vi "LoginCopia2.vi"() -> ()   [LabVIEW 2025]
uses:
  <vilib>/Utility/NIReport.llb/Report Type.ctl
  <vilib>/MakerHub/LINX/Public/Peripherals/Digital/Digital Read 1 Chan.vi
  <vilib>/MakerHub/LINX/Public/Peripherals/Digital/Digital Write 1 Chan.vi
  <vilib>/MakerHub/LINX/Public/Peripherals/Digital/Digital Read N Chans.vi
  <vilib>/MakerHub/LINX/Public/Peripherals/Digital/Digital Write N Chans.vi
  <vilib>/MakerHub/LINX/Private/Local IO/LinxDigitalRead.vi
  <vilib>/MakerHub/LINX/Public/Utilities/Check Channel.vi
  <vilib>/MakerHub/LINX/Private/Local IO/LinxDigitalWrite.vi
  <vilib>/MakerHub/LINX/Public/Utilities/Open Serial.vi
  <vilib>/addons/_office/excel.llb/Excel Easy Table (str).vi
  <vilib>/MakerHub/LINX/Private/Utilties/Generate Error.vi
  <vilib>/Utility/NIReport.llb/NI_report.lvclass
  <vilib>/MakerHub/LINX/LMH-LINX.lvlib
  <vilib>/Utility/NIReport.llb/NI_ReportGenerationCore.lvlib
  <vilib>/addons/_office/NI_ReportGenerationToolkit.lvlib
  <vilib>/Utility/NIReport.llb/Excel/NI_Excel.lvclass
panel:
  in  "stop":bool
  in  "Tab Control":enum32{"Inicio", "Sistema"}(tab)
  in  "Open Button 2":bool
  in  "Contraseña":string
  in  "Usuario":string
  out "Led 1":bool
  out "Led 2":bool
  out "Led 3":bool
  out "Led 4":bool
  out "Led 5":bool
  out "Pin2":dbl
  out "Pin3":dbl
  out "Pin4":dbl
  out "Pin5":dbl
  out "Pin6":dbl
  in  "Puerto Serial":refnum<visa-resource-name>="N/A"
  in  "Secuencia":dbl
  out "Contenido":dbl
  in  "Detener":bool
  in  "Registro Excel":path
  in  "stop 4":bool
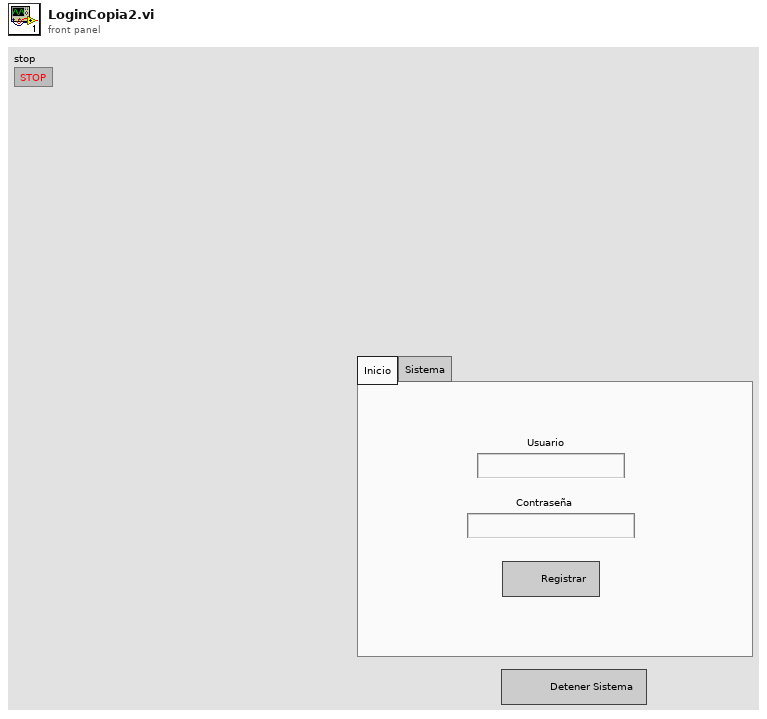
[diagram p1: front panel]
types:
  T1 = typedef "NI_ReportGenerationCore.lvlib/Report Type.ctl" = enum16{"HTML", "Word", "Excel"}
  T2 = typedef "LMH-LINX.lvlib/LINX Ref.ctl" = cluster{"IO":T3, "Interface":T4, "LINX Device Config":T5}
  T3 = typedef "LMH-LINX.lvlib/Platform.ctl" = enum16{"Remote", "Local"}
  T4 = typedef "LMH-LINX.lvlib/Interface.ctl" = enum16{"Serial", "TCP"}
  T5 = typedef "LMH-LINX.lvlib/Device.lvlib/LINX Device Config.ctl" = cluster{"Interface":T4, "COM Port":refnum<visa-resource-name>, "TCP Configuration":T6, "Device Family":u8, "Device ID":u8, "Device Name":string, "TCP Ref":refnum<k5>, "Channels":T7}
  T6 = typedef "LMH-LINX.lvlib/Device.lvlib/TCP Config.ctl" = cluster{"IP Address":string, "Port":u16}
  T7 = typedef "LMH-LINX.lvlib/Channels.ctl" = cluster{"DI":u8[], "DO":u8[], "AI":u8[], "AO":u8[], "PWM":u8[], "QE":u8[], "UART":u8[], "I2C 2":u8[], "SPI":u8[], "CAN":u8[], "Servo":u8[], "AI Ref (V)":dbl, "AI Resolution (Bits)":u8, "AO Ref (V)":dbl, "AO Resolution (Bits)":u8}
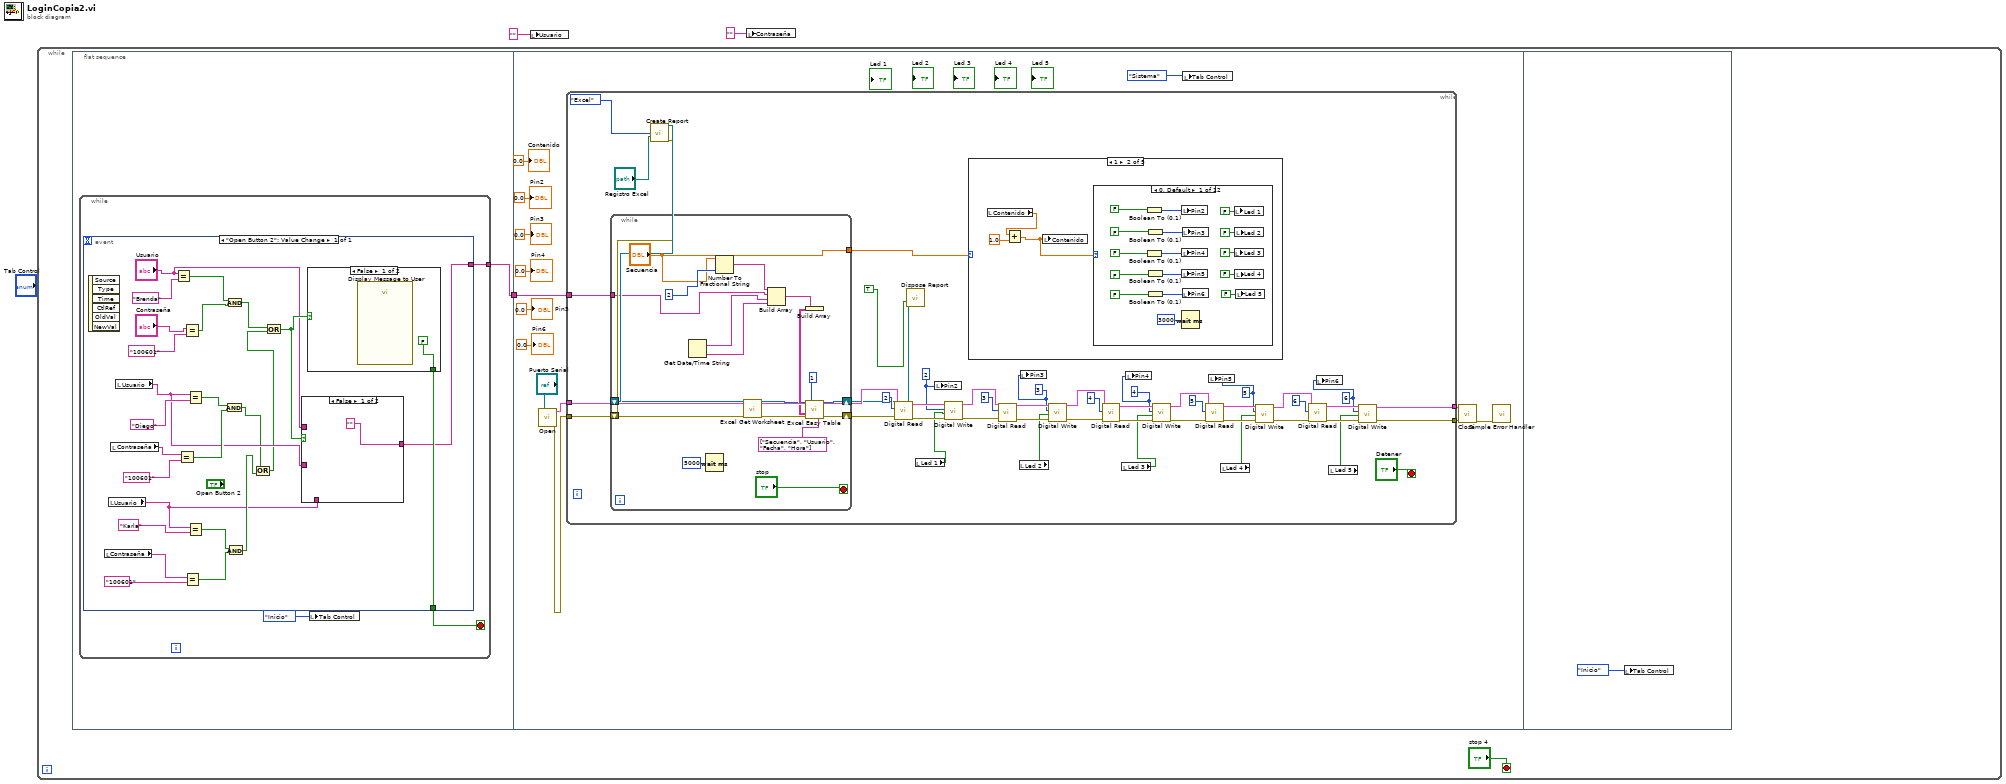
[diagram p0: block diagram]
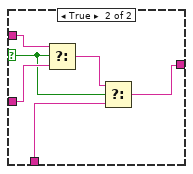
[diagram p2: hidden frame]
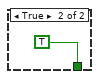
[diagram p3: hidden frame]
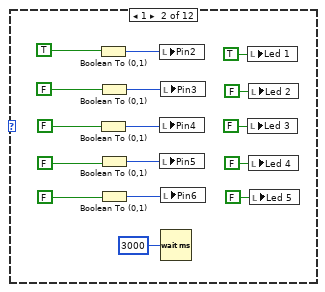
[diagram p5: hidden frame]
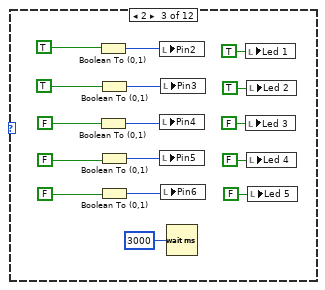
[diagram p6: hidden frame]
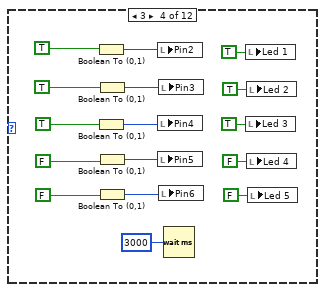
[diagram p7: hidden frame]
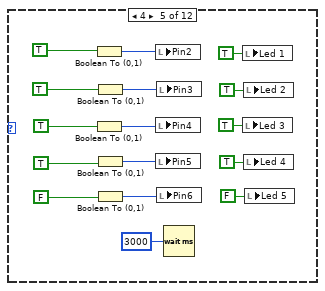
[diagram p8: hidden frame]
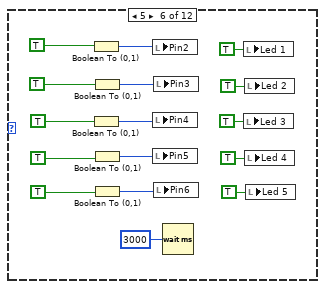
[diagram p9: hidden frame]
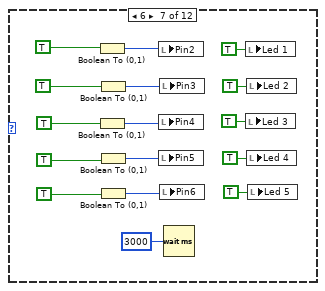
[diagram p10: hidden frame]
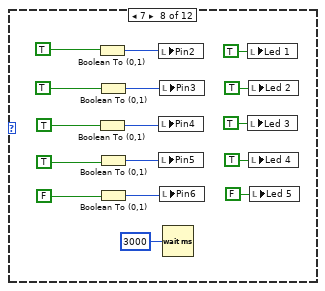
[diagram p11: hidden frame]
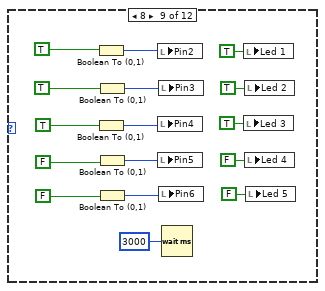
[diagram p12: hidden frame]
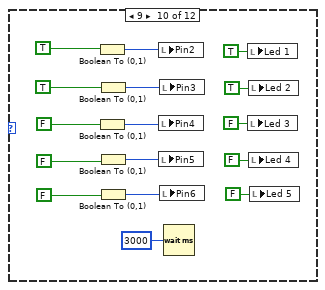
[diagram p13: hidden frame]
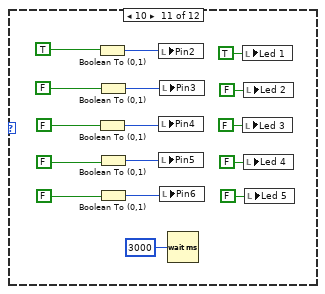
[diagram p14: hidden frame]
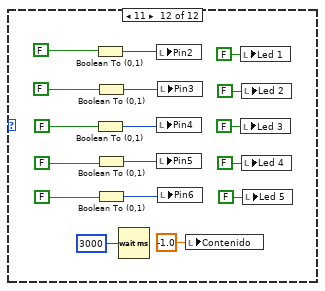
[diagram p15: hidden frame]
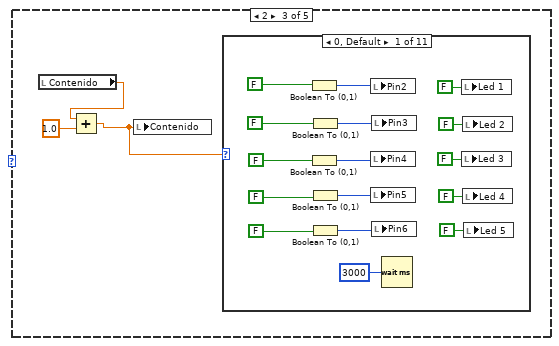
[diagram p16: hidden frame]
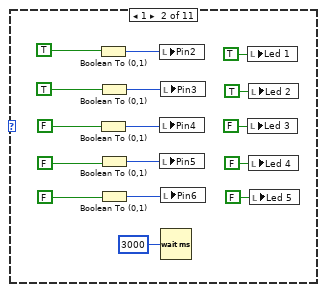
[diagram p17: hidden frame]
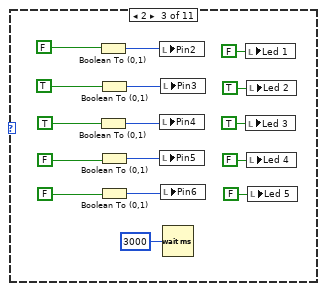
[diagram p18: hidden frame]
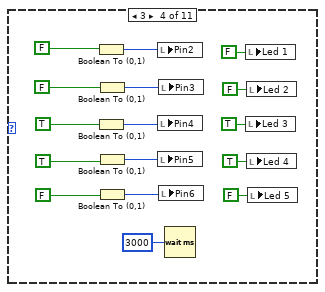
[diagram p19: hidden frame]
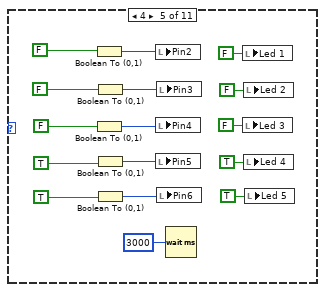
[diagram p20: hidden frame]
diagram:
  n1 = while {
    stop <- "stop 4" stop-if-true
    n2 = flat-sequence {
      tunnel: [w5] -> w3
      tunnel: w3 -> [w43]
      frame #0 {
        n3 = while {
          tunnel: [w6] -> w5
          stop <- w8 stop-if-true
          n4 = event shown="[0] \"Open Button 2\": Value Change" {
            selector: _ -> [_]
            dyn-events: _ -> [_]
            timeout: _ -> [_]
            tunnel: [w33] -> w8
            tunnel: [w18] -> w6
            event "Open Button 2": Value Change {
              n5 = event-data() -> ()  [unwired: 1 in, 6 out]
              n6 = local read "Contraseña"() -> (w16:string)
              n7 = local read "Usuario"() -> (w9:string)
              n8 = local read "Contraseña"() -> (w27:string)
              n9 = local read "Usuario"() -> (w19:string)
              n10 = Equal?(x="Usuario", y="Brenda") -> (x = y?=w23:bool)
              n11 = Equal?(x=w27, y="100601") -> (x = y?=w25:bool)
              n12 = Equal?(x="Contraseña", y="100601") -> (x = y?=w30:bool)
              n13 = Equal?(x=w16, y="100601") -> (x = y?=w13:bool)
              n14 = Equal?(x=w19, y="Diego") -> (x = y?=w26:bool)
              n15 = Equal?(x=w9, y="Karla") -> (x = y?=w14:bool)
              n16 = And(x=w26, y=w25) -> (x .and. y?=w11:bool)
              n17 = And(x=w23, y=w30) -> (x .and. y?=w24:bool)
              n18 = And(x=w14, y=w13) -> (x .and. y?=w12:bool)
              n19 = Or(x=w11, y=w12) -> (x .or. y?=w10:bool)
              n20 = Or(x=w24, y=w10) -> (x .or. y?=w21:bool)
              n21 = case shown="False" w21 {
                selector: w21 -> [_ w35]
                tunnel: "Usuario" -> [_ w40]
                tunnel: w19 -> [_ w39]
                tunnel: ["" ("y") w36] -> w18
                tunnel: w9 -> [_ w38]
                frame False {
                }
                frame True {
                  n22 = Select(t=w40, s=w35, f=w39) -> (s? t:f=w37:string)
                  n23 = Select(t=w37, s=w35, f=w38) -> (s? t:f=w36:string)
                }
              }
              n24 = case shown="False" w21 {
                tunnel: [FALSE TRUE] -> w33
                frame False {
                  n25 = call "Display Message to User"() -> ()  [unwired: 10 in, 2 out]
                }
                frame True {
                }
              }
            }
          }
          n26 = local write "Tab Control"(enum32{"Inicio", "Sistema"}."Inicio" ("Tab Control")) -> ()
        }
      }
      frame #1 {
        n27 = call-poly <vilib>:"Open.vi"("Serial Port"="Puerto Serial") -> ("Error Out"=w45:errorcluster, "LINX Resource"=w46:T2)  [unwired: 8 in, 1 out]
        n28 = while {
          tunnel: [w70] -> w48
          tunnel: [w69] -> w47
          tunnel: w46 -> [w68]
          tunnel: w45 -> [w67]
          tunnel: w43 -> [w57]
          stop <- "Detener" stop-if-true
          w71 = u8 6 ("DO Channel")
          w74 = u8 5 ("DO Channel")
          w75 = u8 4 ("DO Channel")
          w80 = u8 3 ("DO Channel")
          w78 = u8 2 ("DO Channel")
          n29 = call <vilib>:"Create Report.vi"("report type"=Report_Type."Excel", "template (empty)"="Registro Excel") -> ("report out"=w63:refnum<class "NI_report.lvclass">, "error out"=w62:errorcluster)  [unwired: 12 in]
          n30 = while {
            shift-right: [w112] -> w61
            shift-left: w63 -> [w116]
            shift-right: [w111] -> w60
            shift-left: w62 -> [w114]
            tunnel: ["Secuencia"] -> w58
            tunnel: w57 -> [w106]
            stop <- "stop" stop-if-true
            n31 = Get Date/Time String() -> (date string=w105:string, time string=w104:string)  [unwired: 3 in]
            n32 = Wait (ms)(milliseconds to wait=u32 5000) -> ()  [unwired: 1 out]
            n33 = Number To Fractional String(number="Secuencia", precision (6)=i16 2) -> (F-format string=w120:string)  [unwired: 2 in]
            n34 = call <vilib>:"Excel Get Worksheet.vi"("report in"=w116, "error in (no error)"=w114) -> ("report out"=w115:refnum<class "NI_report.lvclass">, "error out"=w113:errorcluster)  [unwired: 12 in]
            n35 = Build Array(w120, w106, w105, w104) -> (w119:string[])
            n36 = Build Array(w119) -> (w118:string[][])
            n37 = call-poly <vilib>:"Excel Easy Table.vi"("report in"=w115, "iteration"=1, "text data"=w118, "error in (no error)"=w113, "column headers"=string[] ["Secuencia", "Usuario", "Fecha", "Hora"]) -> ("report out"=w112:refnum<class "NI_report.lvclass">, "error out"=w111:errorcluster)  [unwired: 6 in, 3 out]
          }
          n38 = call-poly <vilib>:"Digital Read.vi"("Error In"=w67, "DI Channel"=u8 2, "LINX Resource"=w68) -> ("Error Out"=w89:errorcluster, "LINX Resource"=w98:T2)  [unwired: 6 in, 1 out]
          n39 = call-dynamic "Dispose Report.vi"("report in"=w61, "save changes? (F)"=TRUE, "error in (no error)"=w60) -> ()  [unwired: 12 in, 1 out]
          n40 = local read "Led 1"() -> (w79:bool)
          n41 = local write "Pin2"(w78) -> ()
          n42 = call-poly <vilib>:"Digital Write.vi"("Error In"=w89, "Output Value"=w79, "DO Channel"=w78, "LINX Resource"=w98) -> ("Error Out"=w88:errorcluster, "LINX Resource"=w97:T2)  [unwired: 6 in]
          n43 = case shown="1" w58 {
            frame 0, Default {
            }
            frame 1 {
              n44 = local read "Contenido"() -> (w123:dbl)
              n45 = Add(x=w123, y=1.0) -> (x+y=w122:dbl)
              n46 = local write "Contenido"(w122) -> ()
              n47 = case shown="0, Default" w122 {
                frame 0, Default {
                  n48 = Boolean To (0,1)(Boolean=FALSE) -> (0, 1=w140:i16)
                  n49 = Boolean To (0,1)(Boolean=FALSE) -> (0, 1=w138:i16)
                  n50 = Boolean To (0,1)(Boolean=FALSE) -> (0, 1=w139:i16)
                  n51 = Boolean To (0,1)(Boolean=FALSE) -> (0, 1=w137:i16)
                  n52 = Boolean To (0,1)(Boolean=FALSE) -> (0, 1=w136:i16)
                  n53 = local write "Pin2"(w140) -> ()
                  n54 = local write "Pin4"(w138) -> ()
                  n55 = local write "Pin5"(w137) -> ()
                  n56 = Wait (ms)(milliseconds to wait=u32 3000 ("millisecond timer value")) -> ()  [unwired: 1 out]
                  n57 = local write "Pin3"(w139) -> ()
                  n58 = local write "Pin6"(w136) -> ()
                  n59 = local write "Led 1"(FALSE ("Led 1")) -> ()
                  n60 = local write "Led 3"(FALSE ("Led 3")) -> ()
                  n61 = local write "Led 2"(FALSE ("Led 2")) -> ()
                  n62 = local write "Led 4"(FALSE ("Led 4")) -> ()
                  n63 = local write "Led 5"(FALSE ("Led 5")) -> ()
                }
                frame 1 {
                  n64 = Boolean To (0,1)(Boolean=TRUE) -> (0, 1=w155:i16)
                  n65 = Boolean To (0,1)(Boolean=FALSE) -> (0, 1=w151:i16)
                  n66 = Boolean To (0,1)(Boolean=FALSE) -> (0, 1=w153:i16)
                  n67 = Boolean To (0,1)(Boolean=FALSE) -> (0, 1=w149:i16)
                  n68 = Boolean To (0,1)(Boolean=FALSE) -> (0, 1=w147:i16)
                  n69 = local write "Pin2"(w155) -> ()
                  n70 = local write "Pin4"(w151) -> ()
                  n71 = local write "Pin5"(w149) -> ()
                  n72 = local write "Pin3"(w153) -> ()
                  n73 = local write "Pin6"(w147) -> ()
                  n74 = Wait (ms)(milliseconds to wait=u32 3000 ("millisecond timer value")) -> ()  [unwired: 1 out]
                  n75 = local write "Led 1"(TRUE ("Led 1")) -> ()
                  n76 = local write "Led 3"(FALSE ("Led 3")) -> ()
                  n77 = local write "Led 2"(FALSE ("Led 2")) -> ()
                  n78 = local write "Led 4"(FALSE ("Led 4")) -> ()
                  n79 = local write "Led 5"(FALSE ("Led 5")) -> ()
                }
                frame 2 {
                  n80 = Boolean To (0,1)(Boolean=TRUE) -> (0, 1=w172:i16)
                  n81 = Boolean To (0,1)(Boolean=FALSE) -> (0, 1=w170:i16)
                  n82 = Boolean To (0,1)(Boolean=TRUE) -> (0, 1=w171:i16)
                  n83 = Boolean To (0,1)(Boolean=FALSE) -> (0, 1=w169:i16)
                  n84 = Boolean To (0,1)(Boolean=FALSE) -> (0, 1=w168:i16)
                  n85 = local write "Pin2"(w172) -> ()
                  n86 = local write "Pin4"(w170) -> ()
                  n87 = local write "Pin5"(w169) -> ()
                  n88 = local write "Pin3"(w171) -> ()
                  n89 = local write "Pin6"(w168) -> ()
                  n90 = Wait (ms)(milliseconds to wait=u32 3000 ("millisecond timer value")) -> ()  [unwired: 1 out]
                  n91 = local write "Led 1"(TRUE ("Led 1")) -> ()
                  n92 = local write "Led 3"(FALSE ("Led 3")) -> ()
                  n93 = local write "Led 2"(TRUE ("Led 2")) -> ()
                  n94 = local write "Led 4"(FALSE ("Led 4")) -> ()
                  n95 = local write "Led 5"(FALSE ("Led 5")) -> ()
                }
                frame 3 {
                  n96 = Boolean To (0,1)(Boolean=TRUE) -> (0, 1=w188:i16)
                  n97 = Boolean To (0,1)(Boolean=TRUE) -> (0, 1=w186:i16)
                  n98 = Boolean To (0,1)(Boolean=TRUE) -> (0, 1=w187:i16)
                  n99 = Boolean To (0,1)(Boolean=FALSE) -> (0, 1=w185:i16)
                  n100 = Boolean To (0,1)(Boolean=FALSE) -> (0, 1=w184:i16)
                  n101 = local write "Pin2"(w188) -> ()
                  n102 = local write "Pin4"(w186) -> ()
                  n103 = local write "Pin5"(w185) -> ()
                  n104 = local write "Pin3"(w187) -> ()
                  n105 = local write "Pin6"(w184) -> ()
                  n106 = Wait (ms)(milliseconds to wait=u32 3000 ("millisecond timer value")) -> ()  [unwired: 1 out]
                  n107 = local write "Led 1"(TRUE ("Led 1")) -> ()
                  n108 = local write "Led 3"(TRUE ("Led 3")) -> ()
                  n109 = local write "Led 2"(TRUE ("Led 2")) -> ()
                  n110 = local write "Led 4"(FALSE ("Led 4")) -> ()
                  n111 = local write "Led 5"(FALSE ("Led 5")) -> ()
                }
                frame 4 {
                  n112 = Boolean To (0,1)(Boolean=TRUE) -> (0, 1=w204:i16)
                  n113 = Boolean To (0,1)(Boolean=TRUE) -> (0, 1=w202:i16)
                  n114 = Boolean To (0,1)(Boolean=TRUE) -> (0, 1=w203:i16)
                  n115 = Boolean To (0,1)(Boolean=TRUE) -> (0, 1=w201:i16)
                  n116 = Boolean To (0,1)(Boolean=FALSE) -> (0, 1=w200:i16)
                  n117 = local write "Pin2"(w204) -> ()
                  n118 = local write "Pin4"(w202) -> ()
                  n119 = local write "Pin5"(w201) -> ()
                  n120 = local write "Pin3"(w203) -> ()
                  n121 = local write "Pin6"(w200) -> ()
                  n122 = Wait (ms)(milliseconds to wait=u32 3000 ("millisecond timer value")) -> ()  [unwired: 1 out]
                  n123 = local write "Led 1"(TRUE ("Led 1")) -> ()
                  n124 = local write "Led 3"(TRUE ("Led 3")) -> ()
                  n125 = local write "Led 2"(TRUE ("Led 2")) -> ()
                  n126 = local write "Led 4"(TRUE ("Led 4")) -> ()
                  n127 = local write "Led 5"(FALSE ("Led 5")) -> ()
                }
                frame 5 {
                  n128 = Boolean To (0,1)(Boolean=TRUE) -> (0, 1=w220:i16)
                  n129 = Boolean To (0,1)(Boolean=TRUE) -> (0, 1=w218:i16)
                  n130 = Boolean To (0,1)(Boolean=TRUE) -> (0, 1=w219:i16)
                  n131 = Boolean To (0,1)(Boolean=TRUE) -> (0, 1=w217:i16)
                  n132 = Boolean To (0,1)(Boolean=TRUE) -> (0, 1=w216:i16)
                  n133 = local write "Pin2"(w220) -> ()
                  n134 = local write "Pin4"(w218) -> ()
                  n135 = local write "Pin5"(w217) -> ()
                  n136 = local write "Pin3"(w219) -> ()
                  n137 = local write "Pin6"(w216) -> ()
                  n138 = Wait (ms)(milliseconds to wait=u32 3000 ("millisecond timer value")) -> ()  [unwired: 1 out]
                  n139 = local write "Led 1"(TRUE ("Led 1")) -> ()
                  n140 = local write "Led 3"(TRUE ("Led 3")) -> ()
                  n141 = local write "Led 2"(TRUE ("Led 2")) -> ()
                  n142 = local write "Led 4"(TRUE ("Led 4")) -> ()
                  n143 = local write "Led 5"(TRUE ("Led 5")) -> ()
                }
                frame 6 {
                  n144 = Boolean To (0,1)(Boolean=TRUE) -> (0, 1=w236:i16)
                  n145 = Boolean To (0,1)(Boolean=TRUE) -> (0, 1=w234:i16)
                  n146 = Boolean To (0,1)(Boolean=TRUE) -> (0, 1=w235:i16)
                  n147 = Boolean To (0,1)(Boolean=TRUE) -> (0, 1=w233:i16)
                  n148 = Boolean To (0,1)(Boolean=TRUE) -> (0, 1=w232:i16)
                  n149 = local write "Pin2"(w236) -> ()
                  n150 = local write "Pin4"(w234) -> ()
                  n151 = local write "Pin5"(w233) -> ()
                  n152 = local write "Pin3"(w235) -> ()
                  n153 = local write "Pin6"(w232) -> ()
                  n154 = Wait (ms)(milliseconds to wait=u32 3000 ("millisecond timer value")) -> ()  [unwired: 1 out]
                  n155 = local write "Led 1"(TRUE ("Led 1")) -> ()
                  n156 = local write "Led 3"(TRUE ("Led 3")) -> ()
                  n157 = local write "Led 2"(TRUE ("Led 2")) -> ()
                  n158 = local write "Led 4"(TRUE ("Led 4")) -> ()
                  n159 = local write "Led 5"(TRUE ("Led 5")) -> ()
                }
                frame 7 {
                  n160 = Boolean To (0,1)(Boolean=TRUE) -> (0, 1=w252:i16)
                  n161 = Boolean To (0,1)(Boolean=TRUE) -> (0, 1=w250:i16)
                  n162 = Boolean To (0,1)(Boolean=TRUE) -> (0, 1=w251:i16)
                  n163 = Boolean To (0,1)(Boolean=TRUE) -> (0, 1=w249:i16)
                  n164 = Boolean To (0,1)(Boolean=FALSE) -> (0, 1=w248:i16)
                  n165 = local write "Pin2"(w252) -> ()
                  n166 = local write "Pin4"(w250) -> ()
                  n167 = local write "Pin5"(w249) -> ()
                  n168 = local write "Pin3"(w251) -> ()
                  n169 = local write "Pin6"(w248) -> ()
                  n170 = Wait (ms)(milliseconds to wait=u32 3000 ("millisecond timer value")) -> ()  [unwired: 1 out]
                  n171 = local write "Led 1"(TRUE ("Led 1")) -> ()
                  n172 = local write "Led 3"(TRUE ("Led 3")) -> ()
                  n173 = local write "Led 2"(TRUE ("Led 2")) -> ()
                  n174 = local write "Led 4"(TRUE ("Led 4")) -> ()
                  n175 = local write "Led 5"(FALSE ("Led 5")) -> ()
                }
                frame 8 {
                  n176 = Boolean To (0,1)(Boolean=TRUE) -> (0, 1=w268:i16)
                  n177 = Boolean To (0,1)(Boolean=TRUE) -> (0, 1=w266:i16)
                  n178 = Boolean To (0,1)(Boolean=TRUE) -> (0, 1=w267:i16)
                  n179 = Boolean To (0,1)(Boolean=FALSE) -> (0, 1=w265:i16)
                  n180 = Boolean To (0,1)(Boolean=FALSE) -> (0, 1=w264:i16)
                  n181 = local write "Pin2"(w268) -> ()
                  n182 = local write "Pin4"(w266) -> ()
                  n183 = local write "Pin5"(w265) -> ()
                  n184 = local write "Pin3"(w267) -> ()
                  n185 = local write "Pin6"(w264) -> ()
                  n186 = Wait (ms)(milliseconds to wait=u32 3000 ("millisecond timer value")) -> ()  [unwired: 1 out]
                  n187 = local write "Led 1"(TRUE ("Led 1")) -> ()
                  n188 = local write "Led 3"(TRUE ("Led 3")) -> ()
                  n189 = local write "Led 2"(TRUE ("Led 2")) -> ()
                  n190 = local write "Led 4"(FALSE ("Led 4")) -> ()
                  n191 = local write "Led 5"(FALSE ("Led 5")) -> ()
                }
                frame 9 {
                  n192 = Boolean To (0,1)(Boolean=TRUE) -> (0, 1=w284:i16)
                  n193 = Boolean To (0,1)(Boolean=FALSE) -> (0, 1=w282:i16)
                  n194 = Boolean To (0,1)(Boolean=TRUE) -> (0, 1=w283:i16)
                  n195 = Boolean To (0,1)(Boolean=FALSE) -> (0, 1=w281:i16)
                  n196 = Boolean To (0,1)(Boolean=FALSE) -> (0, 1=w280:i16)
                  n197 = local write "Pin2"(w284) -> ()
                  n198 = local write "Pin4"(w282) -> ()
                  n199 = local write "Pin5"(w281) -> ()
                  n200 = local write "Pin3"(w283) -> ()
                  n201 = local write "Pin6"(w280) -> ()
                  n202 = Wait (ms)(milliseconds to wait=u32 3000 ("millisecond timer value")) -> ()  [unwired: 1 out]
                  n203 = local write "Led 1"(TRUE ("Led 1")) -> ()
                  n204 = local write "Led 3"(FALSE ("Led 3")) -> ()
                  n205 = local write "Led 2"(TRUE ("Led 2")) -> ()
                  n206 = local write "Led 4"(FALSE ("Led 4")) -> ()
                  n207 = local write "Led 5"(FALSE ("Led 5")) -> ()
                }
                frame 10 {
                  n208 = Boolean To (0,1)(Boolean=TRUE) -> (0, 1=w300:i16)
                  n209 = Boolean To (0,1)(Boolean=FALSE) -> (0, 1=w298:i16)
                  n210 = Boolean To (0,1)(Boolean=FALSE) -> (0, 1=w299:i16)
                  n211 = Boolean To (0,1)(Boolean=FALSE) -> (0, 1=w297:i16)
                  n212 = Boolean To (0,1)(Boolean=FALSE) -> (0, 1=w296:i16)
                  n213 = local write "Pin2"(w300) -> ()
                  n214 = local write "Pin4"(w298) -> ()
                  n215 = local write "Pin5"(w297) -> ()
                  n216 = local write "Pin3"(w299) -> ()
                  n217 = local write "Pin6"(w296) -> ()
                  n218 = Wait (ms)(milliseconds to wait=u32 3000 ("millisecond timer value")) -> ()  [unwired: 1 out]
                  n219 = local write "Led 1"(TRUE ("Led 1")) -> ()
                  n220 = local write "Led 3"(FALSE ("Led 3")) -> ()
                  n221 = local write "Led 2"(FALSE ("Led 2")) -> ()
                  n222 = local write "Led 4"(FALSE ("Led 4")) -> ()
                  n223 = local write "Led 5"(FALSE ("Led 5")) -> ()
                }
                frame 11 {
                  n224 = Boolean To (0,1)(Boolean=FALSE) -> (0, 1=w317:i16)
                  n225 = Boolean To (0,1)(Boolean=FALSE) -> (0, 1=w315:i16)
                  n226 = Boolean To (0,1)(Boolean=FALSE) -> (0, 1=w316:i16)
                  n227 = Boolean To (0,1)(Boolean=FALSE) -> (0, 1=w314:i16)
                  n228 = Boolean To (0,1)(Boolean=FALSE) -> (0, 1=w313:i16)
                  n229 = Wait (ms)(milliseconds to wait=u32 3000 ("millisecond timer value")) -> ()  [unwired: 1 out]
                  n230 = local write "Pin2"(w317) -> ()
                  n231 = local write "Pin4"(w315) -> ()
                  n232 = local write "Pin5"(w314) -> ()
                  n233 = local write "Pin3"(w316) -> ()
                  n234 = local write "Pin6"(w313) -> ()
                  n235 = local write "Contenido"(-1.0 ("Contenido")) -> ()
                  n236 = local write "Led 1"(FALSE ("Led 1")) -> ()
                  n237 = local write "Led 3"(FALSE ("Led 3")) -> ()
                  n238 = local write "Led 2"(FALSE ("Led 2")) -> ()
                  n239 = local write "Led 4"(FALSE ("Led 4")) -> ()
                  n240 = local write "Led 5"(FALSE ("Led 5")) -> ()
                }
              }
            }
            frame 2 {
              n241 = local read "Contenido"() -> (w320:dbl)
              n242 = Add(x=w320, y=1.0) -> (x+y=w319:dbl)
              n243 = local write "Contenido"(w319) -> ()
              n244 = case shown="0, Default" w319 {
                frame 0, Default {
                  n245 = Boolean To (0,1)(Boolean=FALSE) -> (0, 1=w336:i16)
                  n246 = Boolean To (0,1)(Boolean=FALSE) -> (0, 1=w334:i16)
                  n247 = Boolean To (0,1)(Boolean=FALSE) -> (0, 1=w335:i16)
                  n248 = Boolean To (0,1)(Boolean=FALSE) -> (0, 1=w333:i16)
                  n249 = Boolean To (0,1)(Boolean=FALSE) -> (0, 1=w332:i16)
                  n250 = local write "Pin2"(w336) -> ()
                  n251 = local write "Pin4"(w334) -> ()
                  n252 = local write "Pin5"(w333) -> ()
                  n253 = local write "Pin3"(w335) -> ()
                  n254 = local write "Pin6"(w332) -> ()
                  n255 = Wait (ms)(milliseconds to wait=u32 3000 ("millisecond timer value")) -> ()  [unwired: 1 out]
                  n256 = local write "Led 1"(FALSE ("Led 1")) -> ()
                  n257 = local write "Led 3"(FALSE ("Led 3")) -> ()
                  n258 = local write "Led 2"(FALSE ("Led 2")) -> ()
                  n259 = local write "Led 4"(FALSE ("Led 4")) -> ()
                  n260 = local write "Led 5"(FALSE ("Led 5")) -> ()
                }
                frame 1 {
                  n261 = Boolean To (0,1)(Boolean=TRUE) -> (0, 1=w351:i16)
                  n262 = Boolean To (0,1)(Boolean=FALSE) -> (0, 1=w347:i16)
                  n263 = Boolean To (0,1)(Boolean=TRUE) -> (0, 1=w349:i16)
                  n264 = Boolean To (0,1)(Boolean=FALSE) -> (0, 1=w345:i16)
                  n265 = Boolean To (0,1)(Boolean=FALSE) -> (0, 1=w343:i16)
                  n266 = local write "Pin2"(w351) -> ()
                  n267 = local write "Pin4"(w347) -> ()
                  n268 = local write "Pin5"(w345) -> ()
                  n269 = local write "Pin3"(w349) -> ()
                  n270 = local write "Pin6"(w343) -> ()
                  n271 = Wait (ms)(milliseconds to wait=u32 3000 ("millisecond timer value")) -> ()  [unwired: 1 out]
                  n272 = local write "Led 1"(TRUE ("Led 1")) -> ()
                  n273 = local write "Led 3"(FALSE ("Led 3")) -> ()
                  n274 = local write "Led 2"(TRUE ("Led 2")) -> ()
                  n275 = local write "Led 4"(FALSE ("Led 4")) -> ()
                  n276 = local write "Led 5"(FALSE ("Led 5")) -> ()
                }
                frame 2 {
                  n277 = Boolean To (0,1)(Boolean=FALSE) -> (0, 1=w368:i16)
                  n278 = Boolean To (0,1)(Boolean=TRUE) -> (0, 1=w366:i16)
                  n279 = Boolean To (0,1)(Boolean=TRUE) -> (0, 1=w367:i16)
                  n280 = Boolean To (0,1)(Boolean=FALSE) -> (0, 1=w365:i16)
                  n281 = Boolean To (0,1)(Boolean=FALSE) -> (0, 1=w364:i16)
                  n282 = local write "Pin2"(w368) -> ()
                  n283 = local write "Pin4"(w366) -> ()
                  n284 = local write "Pin5"(w365) -> ()
                  n285 = local write "Pin3"(w367) -> ()
                  n286 = local write "Pin6"(w364) -> ()
                  n287 = Wait (ms)(milliseconds to wait=u32 3000 ("millisecond timer value")) -> ()  [unwired: 1 out]
                  n288 = local write "Led 1"(FALSE ("Led 1")) -> ()
                  n289 = local write "Led 3"(TRUE ("Led 3")) -> ()
                  n290 = local write "Led 2"(TRUE ("Led 2")) -> ()
                  n291 = local write "Led 4"(FALSE ("Led 4")) -> ()
                  n292 = local write "Led 5"(FALSE ("Led 5")) -> ()
                }
                frame 3 {
                  n293 = Boolean To (0,1)(Boolean=FALSE) -> (0, 1=w384:i16)
                  n294 = Boolean To (0,1)(Boolean=TRUE) -> (0, 1=w382:i16)
                  n295 = Boolean To (0,1)(Boolean=FALSE) -> (0, 1=w383:i16)
                  n296 = Boolean To (0,1)(Boolean=TRUE) -> (0, 1=w381:i16)
                  n297 = Boolean To (0,1)(Boolean=FALSE) -> (0, 1=w380:i16)
                  n298 = local write "Pin2"(w384) -> ()
                  n299 = local write "Pin4"(w382) -> ()
                  n300 = local write "Pin5"(w381) -> ()
                  n301 = local write "Pin3"(w383) -> ()
                  n302 = local write "Pin6"(w380) -> ()
                  n303 = Wait (ms)(milliseconds to wait=u32 3000 ("millisecond timer value")) -> ()  [unwired: 1 out]
                  n304 = local write "Led 1"(FALSE ("Led 1")) -> ()
                  n305 = local write "Led 3"(TRUE ("Led 3")) -> ()
                  n306 = local write "Led 2"(FALSE ("Led 2")) -> ()
                  n307 = local write "Led 4"(TRUE ("Led 4")) -> ()
                  n308 = local write "Led 5"(FALSE ("Led 5")) -> ()
                }
                frame 4 {
                  n309 = Boolean To (0,1)(Boolean=FALSE) -> (0, 1=w400:i16)
                  n310 = Boolean To (0,1)(Boolean=FALSE) -> (0, 1=w398:i16)
                  n311 = Boolean To (0,1)(Boolean=FALSE) -> (0, 1=w399:i16)
                  n312 = Boolean To (0,1)(Boolean=TRUE) -> (0, 1=w397:i16)
                  n313 = Boolean To (0,1)(Boolean=TRUE) -> (0, 1=w396:i16)
                  n314 = local write "Pin2"(w400) -> ()
                  n315 = local write "Pin4"(w398) -> ()
                  n316 = local write "Pin5"(w397) -> ()
                  n317 = local write "Pin3"(w399) -> ()
                  n318 = local write "Pin6"(w396) -> ()
                  n319 = Wait (ms)(milliseconds to wait=u32 3000 ("millisecond timer value")) -> ()  [unwired: 1 out]
                  n320 = local write "Led 1"(FALSE ("Led 1")) -> ()
                  n321 = local write "Led 3"(FALSE ("Led 3")) -> ()
                  n322 = local write "Led 2"(FALSE ("Led 2")) -> ()
                  n323 = local write "Led 4"(TRUE ("Led 4")) -> ()
                  n324 = local write "Led 5"(TRUE ("Led 5")) -> ()
                }
                frame 5 {
                  n325 = Boolean To (0,1)(Boolean=FALSE) -> (0, 1=w416:i16)
                  n326 = Boolean To (0,1)(Boolean=FALSE) -> (0, 1=w414:i16)
                  n327 = Boolean To (0,1)(Boolean=FALSE) -> (0, 1=w415:i16)
                  n328 = Boolean To (0,1)(Boolean=FALSE) -> (0, 1=w413:i16)
                  n329 = Boolean To (0,1)(Boolean=FALSE) -> (0, 1=w412:i16)
                  n330 = local write "Pin2"(w416) -> ()
                  n331 = local write "Pin4"(w414) -> ()
                  n332 = local write "Pin5"(w413) -> ()
                  n333 = local write "Pin3"(w415) -> ()
                  n334 = local write "Pin6"(w412) -> ()
                  n335 = Wait (ms)(milliseconds to wait=u32 3000 ("millisecond timer value")) -> ()  [unwired: 1 out]
                  n336 = local write "Led 1"(FALSE ("Led 1")) -> ()
                  n337 = local write "Led 3"(FALSE ("Led 3")) -> ()
                  n338 = local write "Led 2"(FALSE ("Led 2")) -> ()
                  n339 = local write "Led 4"(FALSE ("Led 4")) -> ()
                  n340 = local write "Led 5"(FALSE ("Led 5")) -> ()
                }
                frame 6 {
                  n341 = Boolean To (0,1)(Boolean=FALSE) -> (0, 1=w432:i16)
                  n342 = Boolean To (0,1)(Boolean=FALSE) -> (0, 1=w430:i16)
                  n343 = Boolean To (0,1)(Boolean=FALSE) -> (0, 1=w431:i16)
                  n344 = Boolean To (0,1)(Boolean=TRUE) -> (0, 1=w429:i16)
                  n345 = Boolean To (0,1)(Boolean=TRUE) -> (0, 1=w428:i16)
                  n346 = local write "Pin2"(w432) -> ()
                  n347 = local write "Pin4"(w430) -> ()
                  n348 = local write "Pin5"(w429) -> ()
                  n349 = local write "Pin3"(w431) -> ()
                  n350 = local write "Pin6"(w428) -> ()
                  n351 = Wait (ms)(milliseconds to wait=u32 3000 ("millisecond timer value")) -> ()  [unwired: 1 out]
                  n352 = local write "Led 1"(FALSE ("Led 1")) -> ()
                  n353 = local write "Led 3"(FALSE ("Led 3")) -> ()
                  n354 = local write "Led 2"(FALSE ("Led 2")) -> ()
                  n355 = local write "Led 4"(TRUE ("Led 4")) -> ()
                  n356 = local write "Led 5"(TRUE ("Led 5")) -> ()
                }
                frame 7 {
                  n357 = Boolean To (0,1)(Boolean=FALSE) -> (0, 1=w448:i16)
                  n358 = Boolean To (0,1)(Boolean=TRUE) -> (0, 1=w446:i16)
                  n359 = Boolean To (0,1)(Boolean=FALSE) -> (0, 1=w447:i16)
                  n360 = Boolean To (0,1)(Boolean=TRUE) -> (0, 1=w445:i16)
                  n361 = Boolean To (0,1)(Boolean=FALSE) -> (0, 1=w444:i16)
                  n362 = local write "Pin2"(w448) -> ()
                  n363 = local write "Pin4"(w446) -> ()
                  n364 = local write "Pin5"(w445) -> ()
                  n365 = local write "Pin3"(w447) -> ()
                  n366 = local write "Pin6"(w444) -> ()
                  n367 = Wait (ms)(milliseconds to wait=u32 3000 ("millisecond timer value")) -> ()  [unwired: 1 out]
                  n368 = local write "Led 1"(FALSE ("Led 1")) -> ()
                  n369 = local write "Led 3"(TRUE ("Led 3")) -> ()
                  n370 = local write "Led 2"(FALSE ("Led 2")) -> ()
                  n371 = local write "Led 4"(TRUE ("Led 4")) -> ()
                  n372 = local write "Led 5"(FALSE ("Led 5")) -> ()
                }
                frame 8 {
                  n373 = Boolean To (0,1)(Boolean=FALSE) -> (0, 1=w464:i16)
                  n374 = Boolean To (0,1)(Boolean=TRUE) -> (0, 1=w462:i16)
                  n375 = Boolean To (0,1)(Boolean=TRUE) -> (0, 1=w463:i16)
                  n376 = Boolean To (0,1)(Boolean=FALSE) -> (0, 1=w461:i16)
                  n377 = Boolean To (0,1)(Boolean=FALSE) -> (0, 1=w460:i16)
                  n378 = local write "Pin2"(w464) -> ()
                  n379 = local write "Pin4"(w462) -> ()
                  n380 = local write "Pin5"(w461) -> ()
                  n381 = local write "Pin3"(w463) -> ()
                  n382 = local write "Pin6"(w460) -> ()
                  n383 = Wait (ms)(milliseconds to wait=u32 3000 ("millisecond timer value")) -> ()  [unwired: 1 out]
                  n384 = local write "Led 1"(FALSE ("Led 1")) -> ()
                  n385 = local write "Led 3"(TRUE ("Led 3")) -> ()
                  n386 = local write "Led 2"(TRUE ("Led 2")) -> ()
                  n387 = local write "Led 4"(FALSE ("Led 4")) -> ()
                  n388 = local write "Led 5"(FALSE ("Led 5")) -> ()
                }
                frame 9 {
                  n389 = Boolean To (0,1)(Boolean=TRUE) -> (0, 1=w480:i16)
                  n390 = Boolean To (0,1)(Boolean=FALSE) -> (0, 1=w478:i16)
                  n391 = Boolean To (0,1)(Boolean=TRUE) -> (0, 1=w479:i16)
                  n392 = Boolean To (0,1)(Boolean=FALSE) -> (0, 1=w477:i16)
                  n393 = Boolean To (0,1)(Boolean=FALSE) -> (0, 1=w476:i16)
                  n394 = local write "Pin2"(w480) -> ()
                  n395 = local write "Pin4"(w478) -> ()
                  n396 = local write "Pin5"(w477) -> ()
                  n397 = local write "Pin3"(w479) -> ()
                  n398 = local write "Pin6"(w476) -> ()
                  n399 = Wait (ms)(milliseconds to wait=u32 3000 ("millisecond timer value")) -> ()  [unwired: 1 out]
                  n400 = local write "Led 1"(TRUE ("Led 1")) -> ()
                  n401 = local write "Led 3"(FALSE ("Led 3")) -> ()
                  n402 = local write "Led 2"(TRUE ("Led 2")) -> ()
                  n403 = local write "Led 4"(FALSE ("Led 4")) -> ()
                  n404 = local write "Led 5"(FALSE ("Led 5")) -> ()
                }
                frame 10 {
                  n405 = Boolean To (0,1)(Boolean=FALSE) -> (0, 1=w497:i16)
                  n406 = Boolean To (0,1)(Boolean=FALSE) -> (0, 1=w495:i16)
                  n407 = Boolean To (0,1)(Boolean=FALSE) -> (0, 1=w496:i16)
                  n408 = Boolean To (0,1)(Boolean=FALSE) -> (0, 1=w494:i16)
                  n409 = Boolean To (0,1)(Boolean=FALSE) -> (0, 1=w493:i16)
                  n410 = Wait (ms)(milliseconds to wait=u32 3000 ("millisecond timer value")) -> ()  [unwired: 1 out]
                  n411 = local write "Pin2"(w497) -> ()
                  n412 = local write "Pin4"(w495) -> ()
                  n413 = local write "Pin5"(w494) -> ()
                  n414 = local write "Pin3"(w496) -> ()
                  n415 = local write "Pin6"(w493) -> ()
                  n416 = local write "Contenido"(-1.0 ("Contenido")) -> ()
                  n417 = local write "Led 1"(FALSE ("Led 1")) -> ()
                  n418 = local write "Led 3"(FALSE ("Led 3")) -> ()
                  n419 = local write "Led 2"(FALSE ("Led 2")) -> ()
                  n420 = local write "Led 4"(FALSE ("Led 4")) -> ()
                  n421 = local write "Led 5"(FALSE ("Led 5")) -> ()
                }
              }
            }
            frame 3 {
              n422 = local read "Contenido"() -> (w500:dbl)
              n423 = Add(x=w500, y=1.0) -> (x+y=w499:dbl)
              n424 = local write "Contenido"(w499) -> ()
              n425 = case shown="0, Default" w499 {
                frame 0, Default {
                  n426 = Boolean To (0,1)(Boolean=FALSE) -> (0, 1=w516:i16)
                  n427 = Boolean To (0,1)(Boolean=FALSE) -> (0, 1=w514:i16)
                  n428 = Boolean To (0,1)(Boolean=FALSE) -> (0, 1=w515:i16)
                  n429 = Boolean To (0,1)(Boolean=FALSE) -> (0, 1=w513:i16)
                  n430 = Boolean To (0,1)(Boolean=FALSE) -> (0, 1=w512:i16)
                  n431 = local write "Pin2"(w516) -> ()
                  n432 = local write "Pin4"(w514) -> ()
                  n433 = local write "Pin5"(w513) -> ()
                  n434 = local write "Pin3"(w515) -> ()
                  n435 = local write "Pin6"(w512) -> ()
                  n436 = Wait (ms)(milliseconds to wait=u32 3000 ("millisecond timer value")) -> ()  [unwired: 1 out]
                  n437 = local write "Led 1"(FALSE ("Led 1")) -> ()
                  n438 = local write "Led 3"(FALSE ("Led 3")) -> ()
                  n439 = local write "Led 2"(FALSE ("Led 2")) -> ()
                  n440 = local write "Led 4"(FALSE ("Led 4")) -> ()
                  n441 = local write "Led 5"(FALSE ("Led 5")) -> ()
                }
                frame 1 {
                  n442 = Boolean To (0,1)(Boolean=TRUE) -> (0, 1=w531:i16)
                  n443 = Boolean To (0,1)(Boolean=FALSE) -> (0, 1=w527:i16)
                  n444 = Boolean To (0,1)(Boolean=FALSE) -> (0, 1=w529:i16)
                  n445 = Boolean To (0,1)(Boolean=FALSE) -> (0, 1=w525:i16)
                  n446 = Boolean To (0,1)(Boolean=TRUE) -> (0, 1=w523:i16)
                  n447 = local write "Pin2"(w531) -> ()
                  n448 = local write "Pin4"(w527) -> ()
                  n449 = local write "Pin5"(w525) -> ()
                  n450 = local write "Pin3"(w529) -> ()
                  n451 = local write "Pin6"(w523) -> ()
                  n452 = Wait (ms)(milliseconds to wait=u32 3000 ("millisecond timer value")) -> ()  [unwired: 1 out]
                  n453 = local write "Led 1"(TRUE ("Led 1")) -> ()
                  n454 = local write "Led 3"(FALSE ("Led 3")) -> ()
                  n455 = local write "Led 2"(FALSE ("Led 2")) -> ()
                  n456 = local write "Led 4"(FALSE ("Led 4")) -> ()
                  n457 = local write "Led 5"(TRUE ("Led 5")) -> ()
                }
                frame 2 {
                  n458 = Boolean To (0,1)(Boolean=FALSE) -> (0, 1=w548:i16)
                  n459 = Boolean To (0,1)(Boolean=FALSE) -> (0, 1=w546:i16)
                  n460 = Boolean To (0,1)(Boolean=TRUE) -> (0, 1=w547:i16)
                  n461 = Boolean To (0,1)(Boolean=TRUE) -> (0, 1=w545:i16)
                  n462 = Boolean To (0,1)(Boolean=FALSE) -> (0, 1=w544:i16)
                  n463 = local write "Pin2"(w548) -> ()
                  n464 = local write "Pin4"(w546) -> ()
                  n465 = local write "Pin5"(w545) -> ()
                  n466 = local write "Pin3"(w547) -> ()
                  n467 = local write "Pin6"(w544) -> ()
                  n468 = Wait (ms)(milliseconds to wait=u32 3000 ("millisecond timer value")) -> ()  [unwired: 1 out]
                  n469 = local write "Led 1"(FALSE ("Led 1")) -> ()
                  n470 = local write "Led 3"(FALSE ("Led 3")) -> ()
                  n471 = local write "Led 2"(TRUE ("Led 2")) -> ()
                  n472 = local write "Led 4"(TRUE ("Led 4")) -> ()
                  n473 = local write "Led 5"(FALSE ("Led 5")) -> ()
                }
                frame 3 {
                  n474 = Boolean To (0,1)(Boolean=TRUE) -> (0, 1=w564:i16)
                  n475 = Boolean To (0,1)(Boolean=TRUE) -> (0, 1=w562:i16)
                  n476 = Boolean To (0,1)(Boolean=FALSE) -> (0, 1=w563:i16)
                  n477 = Boolean To (0,1)(Boolean=FALSE) -> (0, 1=w561:i16)
                  n478 = Boolean To (0,1)(Boolean=FALSE) -> (0, 1=w560:i16)
                  n479 = local write "Pin2"(w564) -> ()
                  n480 = local write "Pin4"(w562) -> ()
                  n481 = local write "Pin5"(w561) -> ()
                  n482 = local write "Pin3"(w563) -> ()
                  n483 = local write "Pin6"(w560) -> ()
                  n484 = Wait (ms)(milliseconds to wait=u32 3000 ("millisecond timer value")) -> ()  [unwired: 1 out]
                  n485 = local write "Led 1"(TRUE ("Led 1")) -> ()
                  n486 = local write "Led 3"(TRUE ("Led 3")) -> ()
                  n487 = local write "Led 2"(FALSE ("Led 2")) -> ()
                  n488 = local write "Led 4"(FALSE ("Led 4")) -> ()
                  n489 = local write "Led 5"(FALSE ("Led 5")) -> ()
                }
                frame 4 {
                  n490 = Boolean To (0,1)(Boolean=FALSE) -> (0, 1=w580:i16)
                  n491 = Boolean To (0,1)(Boolean=FALSE) -> (0, 1=w578:i16)
                  n492 = Boolean To (0,1)(Boolean=TRUE) -> (0, 1=w579:i16)
                  n493 = Boolean To (0,1)(Boolean=TRUE) -> (0, 1=w577:i16)
                  n494 = Boolean To (0,1)(Boolean=FALSE) -> (0, 1=w576:i16)
                  n495 = local write "Pin2"(w580) -> ()
                  n496 = local write "Pin4"(w578) -> ()
                  n497 = local write "Pin5"(w577) -> ()
                  n498 = local write "Pin3"(w579) -> ()
                  n499 = local write "Pin6"(w576) -> ()
                  n500 = Wait (ms)(milliseconds to wait=u32 3000 ("millisecond timer value")) -> ()  [unwired: 1 out]
                  n501 = local write "Led 1"(FALSE ("Led 1")) -> ()
                  n502 = local write "Led 3"(FALSE ("Led 3")) -> ()
                  n503 = local write "Led 2"(TRUE ("Led 2")) -> ()
                  n504 = local write "Led 4"(TRUE ("Led 4")) -> ()
                  n505 = local write "Led 5"(FALSE ("Led 5")) -> ()
                }
                frame 5 {
                  n506 = Boolean To (0,1)(Boolean=FALSE) -> (0, 1=w596:i16)
                  n507 = Boolean To (0,1)(Boolean=TRUE) -> (0, 1=w594:i16)
                  n508 = Boolean To (0,1)(Boolean=FALSE) -> (0, 1=w595:i16)
                  n509 = Boolean To (0,1)(Boolean=FALSE) -> (0, 1=w593:i16)
                  n510 = Boolean To (0,1)(Boolean=TRUE) -> (0, 1=w592:i16)
                  n511 = local write "Pin2"(w596) -> ()
                  n512 = local write "Pin4"(w594) -> ()
                  n513 = local write "Pin5"(w593) -> ()
                  n514 = local write "Pin3"(w595) -> ()
                  n515 = local write "Pin6"(w592) -> ()
                  n516 = Wait (ms)(milliseconds to wait=u32 3000 ("millisecond timer value")) -> ()  [unwired: 1 out]
                  n517 = local write "Led 1"(FALSE ("Led 1")) -> ()
                  n518 = local write "Led 3"(TRUE ("Led 3")) -> ()
                  n519 = local write "Led 2"(FALSE ("Led 2")) -> ()
                  n520 = local write "Led 4"(FALSE ("Led 4")) -> ()
                  n521 = local write "Led 5"(TRUE ("Led 5")) -> ()
                }
                frame 6 {
                  n522 = Boolean To (0,1)(Boolean=FALSE) -> (0, 1=w612:i16)
                  n523 = Boolean To (0,1)(Boolean=FALSE) -> (0, 1=w610:i16)
                  n524 = Boolean To (0,1)(Boolean=FALSE) -> (0, 1=w611:i16)
                  n525 = Boolean To (0,1)(Boolean=FALSE) -> (0, 1=w609:i16)
                  n526 = Boolean To (0,1)(Boolean=FALSE) -> (0, 1=w608:i16)
                  n527 = local write "Pin2"(w612) -> ()
                  n528 = local write "Pin4"(w610) -> ()
                  n529 = local write "Pin5"(w609) -> ()
                  n530 = local write "Pin3"(w611) -> ()
                  n531 = local write "Pin6"(w608) -> ()
                  n532 = Wait (ms)(milliseconds to wait=u32 3000 ("millisecond timer value")) -> ()  [unwired: 1 out]
                  n533 = local write "Led 1"(FALSE ("Led 1")) -> ()
                  n534 = local write "Led 3"(FALSE ("Led 3")) -> ()
                  n535 = local write "Led 2"(FALSE ("Led 2")) -> ()
                  n536 = local write "Led 4"(FALSE ("Led 4")) -> ()
                  n537 = local write "Led 5"(FALSE ("Led 5")) -> ()
                }
                frame 7 {
                  n538 = Boolean To (0,1)(Boolean=FALSE) -> (0, 1=w628:i16)
                  n539 = Boolean To (0,1)(Boolean=TRUE) -> (0, 1=w626:i16)
                  n540 = Boolean To (0,1)(Boolean=FALSE) -> (0, 1=w627:i16)
                  n541 = Boolean To (0,1)(Boolean=FALSE) -> (0, 1=w625:i16)
                  n542 = Boolean To (0,1)(Boolean=TRUE) -> (0, 1=w624:i16)
                  n543 = local write "Pin2"(w628) -> ()
                  n544 = local write "Pin4"(w626) -> ()
                  n545 = local write "Pin5"(w625) -> ()
                  n546 = local write "Pin3"(w627) -> ()
                  n547 = local write "Pin6"(w624) -> ()
                  n548 = Wait (ms)(milliseconds to wait=u32 3000 ("millisecond timer value")) -> ()  [unwired: 1 out]
                  n549 = local write "Led 1"(FALSE ("Led 1")) -> ()
                  n550 = local write "Led 3"(TRUE ("Led 3")) -> ()
                  n551 = local write "Led 2"(FALSE ("Led 2")) -> ()
                  n552 = local write "Led 4"(FALSE ("Led 4")) -> ()
                  n553 = local write "Led 5"(TRUE ("Led 5")) -> ()
                }
                frame 8 {
                  n554 = Boolean To (0,1)(Boolean=FALSE) -> (0, 1=w644:i16)
                  n555 = Boolean To (0,1)(Boolean=FALSE) -> (0, 1=w642:i16)
                  n556 = Boolean To (0,1)(Boolean=TRUE) -> (0, 1=w643:i16)
                  n557 = Boolean To (0,1)(Boolean=TRUE) -> (0, 1=w641:i16)
                  n558 = Boolean To (0,1)(Boolean=FALSE) -> (0, 1=w640:i16)
                  n559 = local write "Pin2"(w644) -> ()
                  n560 = local write "Pin4"(w642) -> ()
                  n561 = local write "Pin5"(w641) -> ()
                  n562 = local write "Pin3"(w643) -> ()
                  n563 = local write "Pin6"(w640) -> ()
                  n564 = Wait (ms)(milliseconds to wait=u32 3000 ("millisecond timer value")) -> ()  [unwired: 1 out]
                  n565 = local write "Led 1"(FALSE ("Led 1")) -> ()
                  n566 = local write "Led 3"(FALSE ("Led 3")) -> ()
                  n567 = local write "Led 2"(TRUE ("Led 2")) -> ()
                  n568 = local write "Led 4"(TRUE ("Led 4")) -> ()
                  n569 = local write "Led 5"(FALSE ("Led 5")) -> ()
                }
                frame 9 {
                  n570 = Boolean To (0,1)(Boolean=TRUE) -> (0, 1=w660:i16)
                  n571 = Boolean To (0,1)(Boolean=TRUE) -> (0, 1=w658:i16)
                  n572 = Boolean To (0,1)(Boolean=FALSE) -> (0, 1=w659:i16)
                  n573 = Boolean To (0,1)(Boolean=FALSE) -> (0, 1=w657:i16)
                  n574 = Boolean To (0,1)(Boolean=FALSE) -> (0, 1=w656:i16)
                  n575 = local write "Pin2"(w660) -> ()
                  n576 = local write "Pin4"(w658) -> ()
                  n577 = local write "Pin5"(w657) -> ()
                  n578 = local write "Pin3"(w659) -> ()
                  n579 = local write "Pin6"(w656) -> ()
                  n580 = Wait (ms)(milliseconds to wait=u32 3000 ("millisecond timer value")) -> ()  [unwired: 1 out]
                  n581 = local write "Led 1"(TRUE ("Led 1")) -> ()
                  n582 = local write "Led 3"(TRUE ("Led 3")) -> ()
                  n583 = local write "Led 2"(FALSE ("Led 2")) -> ()
                  n584 = local write "Led 4"(FALSE ("Led 4")) -> ()
                  n585 = local write "Led 5"(FALSE ("Led 5")) -> ()
                }
                frame 10 {
                  n586 = Boolean To (0,1)(Boolean=FALSE) -> (0, 1=w676:i16)
                  n587 = Boolean To (0,1)(Boolean=FALSE) -> (0, 1=w674:i16)
                  n588 = Boolean To (0,1)(Boolean=TRUE) -> (0, 1=w675:i16)
                  n589 = Boolean To (0,1)(Boolean=TRUE) -> (0, 1=w673:i16)
                  n590 = Boolean To (0,1)(Boolean=FALSE) -> (0, 1=w672:i16)
                  n591 = local write "Pin2"(w676) -> ()
                  n592 = local write "Pin4"(w674) -> ()
                  n593 = local write "Pin5"(w673) -> ()
                  n594 = local write "Pin3"(w675) -> ()
                  n595 = local write "Pin6"(w672) -> ()
                  n596 = Wait (ms)(milliseconds to wait=u32 3000 ("millisecond timer value")) -> ()  [unwired: 1 out]
                  n597 = local write "Led 1"(FALSE ("Led 1")) -> ()
                  n598 = local write "Led 3"(FALSE ("Led 3")) -> ()
                  n599 = local write "Led 2"(TRUE ("Led 2")) -> ()
                  n600 = local write "Led 4"(TRUE ("Led 4")) -> ()
                  n601 = local write "Led 5"(FALSE ("Led 5")) -> ()
                }
                frame 11 {
                  n602 = Boolean To (0,1)(Boolean=TRUE) -> (0, 1=w692:i16)
                  n603 = Boolean To (0,1)(Boolean=FALSE) -> (0, 1=w690:i16)
                  n604 = Boolean To (0,1)(Boolean=FALSE) -> (0, 1=w691:i16)
                  n605 = Boolean To (0,1)(Boolean=FALSE) -> (0, 1=w689:i16)
                  n606 = Boolean To (0,1)(Boolean=TRUE) -> (0, 1=w688:i16)
                  n607 = local write "Pin2"(w692) -> ()
                  n608 = local write "Pin4"(w690) -> ()
                  n609 = local write "Pin5"(w689) -> ()
                  n610 = local write "Pin3"(w691) -> ()
                  n611 = local write "Pin6"(w688) -> ()
                  n612 = Wait (ms)(milliseconds to wait=u32 3000 ("millisecond timer value")) -> ()  [unwired: 1 out]
                  n613 = local write "Led 1"(TRUE ("Led 1")) -> ()
                  n614 = local write "Led 3"(FALSE ("Led 3")) -> ()
                  n615 = local write "Led 2"(FALSE ("Led 2")) -> ()
                  n616 = local write "Led 4"(FALSE ("Led 4")) -> ()
                  n617 = local write "Led 5"(TRUE ("Led 5")) -> ()
                }
                frame 12 {
                  n618 = Boolean To (0,1)(Boolean=FALSE) -> (0, 1=w709:i16)
                  n619 = Boolean To (0,1)(Boolean=FALSE) -> (0, 1=w707:i16)
                  n620 = Boolean To (0,1)(Boolean=FALSE) -> (0, 1=w708:i16)
                  n621 = Boolean To (0,1)(Boolean=FALSE) -> (0, 1=w706:i16)
                  n622 = Boolean To (0,1)(Boolean=FALSE) -> (0, 1=w705:i16)
                  n623 = Wait (ms)(milliseconds to wait=u32 3000 ("millisecond timer value")) -> ()  [unwired: 1 out]
                  n624 = local write "Pin2"(w709) -> ()
                  n625 = local write "Pin4"(w707) -> ()
                  n626 = local write "Pin5"(w706) -> ()
                  n627 = local write "Pin3"(w708) -> ()
                  n628 = local write "Pin6"(w705) -> ()
                  n629 = local write "Contenido"(-1.0 ("Contenido")) -> ()
                  n630 = local write "Led 1"(FALSE ("Led 1")) -> ()
                  n631 = local write "Led 3"(FALSE ("Led 3")) -> ()
                  n632 = local write "Led 2"(FALSE ("Led 2")) -> ()
                  n633 = local write "Led 4"(FALSE ("Led 4")) -> ()
                  n634 = local write "Led 5"(FALSE ("Led 5")) -> ()
                }
              }
            }
            frame 4 {
              n635 = local read "Contenido"() -> (w712:dbl)
              n636 = Add(x=w712, y=1.0) -> (x+y=w711:dbl)
              n637 = local write "Contenido"(w711) -> ()
              n638 = case shown="0, Default" w711 {
                frame 0, Default {
                  n639 = Boolean To (0,1)(Boolean=FALSE) -> (0, 1=w728:i16)
                  n640 = Boolean To (0,1)(Boolean=FALSE) -> (0, 1=w726:i16)
                  n641 = Boolean To (0,1)(Boolean=FALSE) -> (0, 1=w727:i16)
                  n642 = Boolean To (0,1)(Boolean=FALSE) -> (0, 1=w725:i16)
                  n643 = Boolean To (0,1)(Boolean=FALSE) -> (0, 1=w724:i16)
                  n644 = local write "Pin2"(w728) -> ()
                  n645 = local write "Pin4"(w726) -> ()
                  n646 = local write "Pin5"(w725) -> ()
                  n647 = local write "Pin3"(w727) -> ()
                  n648 = local write "Pin6"(w724) -> ()
                  n649 = Wait (ms)(milliseconds to wait=u32 3000 ("millisecond timer value")) -> ()  [unwired: 1 out]
                  n650 = local write "Led 1"(FALSE ("Led 1")) -> ()
                  n651 = local write "Led 3"(FALSE ("Led 3")) -> ()
                  n652 = local write "Led 2"(FALSE ("Led 2")) -> ()
                  n653 = local write "Led 4"(FALSE ("Led 4")) -> ()
                  n654 = local write "Led 5"(FALSE ("Led 5")) -> ()
                }
                frame 1 {
                  n655 = Boolean To (0,1)(Boolean=TRUE) -> (0, 1=w743:i16)
                  n656 = Boolean To (0,1)(Boolean=FALSE) -> (0, 1=w739:i16)
                  n657 = Boolean To (0,1)(Boolean=FALSE) -> (0, 1=w741:i16)
                  n658 = Boolean To (0,1)(Boolean=FALSE) -> (0, 1=w737:i16)
                  n659 = Boolean To (0,1)(Boolean=FALSE) -> (0, 1=w735:i16)
                  n660 = local write "Pin2"(w743) -> ()
                  n661 = local write "Pin4"(w739) -> ()
                  n662 = local write "Pin5"(w737) -> ()
                  n663 = local write "Pin3"(w741) -> ()
                  n664 = local write "Pin6"(w735) -> ()
                  n665 = Wait (ms)(milliseconds to wait=u32 3000 ("millisecond timer value")) -> ()  [unwired: 1 out]
                  n666 = local write "Led 1"(TRUE ("Led 1")) -> ()
                  n667 = local write "Led 3"(FALSE ("Led 3")) -> ()
                  n668 = local write "Led 2"(FALSE ("Led 2")) -> ()
                  n669 = local write "Led 4"(FALSE ("Led 4")) -> ()
                  n670 = local write "Led 5"(FALSE ("Led 5")) -> ()
                }
                frame 2 {
                  n671 = Boolean To (0,1)(Boolean=FALSE) -> (0, 1=w760:i16)
                  n672 = Boolean To (0,1)(Boolean=FALSE) -> (0, 1=w758:i16)
                  n673 = Boolean To (0,1)(Boolean=FALSE) -> (0, 1=w759:i16)
                  n674 = Boolean To (0,1)(Boolean=TRUE) -> (0, 1=w757:i16)
                  n675 = Boolean To (0,1)(Boolean=FALSE) -> (0, 1=w756:i16)
                  n676 = local write "Pin2"(w760) -> ()
                  n677 = local write "Pin4"(w758) -> ()
                  n678 = local write "Pin5"(w757) -> ()
                  n679 = local write "Pin3"(w759) -> ()
                  n680 = local write "Pin6"(w756) -> ()
                  n681 = Wait (ms)(milliseconds to wait=u32 3000 ("millisecond timer value")) -> ()  [unwired: 1 out]
                  n682 = local write "Led 1"(FALSE ("Led 1")) -> ()
                  n683 = local write "Led 3"(FALSE ("Led 3")) -> ()
                  n684 = local write "Led 2"(FALSE ("Led 2")) -> ()
                  n685 = local write "Led 4"(TRUE ("Led 4")) -> ()
                  n686 = local write "Led 5"(FALSE ("Led 5")) -> ()
                }
                frame 3 {
                  n687 = Boolean To (0,1)(Boolean=FALSE) -> (0, 1=w776:i16)
                  n688 = Boolean To (0,1)(Boolean=TRUE) -> (0, 1=w774:i16)
                  n689 = Boolean To (0,1)(Boolean=FALSE) -> (0, 1=w775:i16)
                  n690 = Boolean To (0,1)(Boolean=FALSE) -> (0, 1=w773:i16)
                  n691 = Boolean To (0,1)(Boolean=FALSE) -> (0, 1=w772:i16)
                  n692 = local write "Pin2"(w776) -> ()
                  n693 = local write "Pin4"(w774) -> ()
                  n694 = local write "Pin5"(w773) -> ()
                  n695 = local write "Pin3"(w775) -> ()
                  n696 = local write "Pin6"(w772) -> ()
                  n697 = Wait (ms)(milliseconds to wait=u32 3000 ("millisecond timer value")) -> ()  [unwired: 1 out]
                  n698 = local write "Led 1"(FALSE ("Led 1")) -> ()
                  n699 = local write "Led 3"(TRUE ("Led 3")) -> ()
                  n700 = local write "Led 2"(FALSE ("Led 2")) -> ()
                  n701 = local write "Led 4"(FALSE ("Led 4")) -> ()
                  n702 = local write "Led 5"(FALSE ("Led 5")) -> ()
                }
                frame 4 {
                  n703 = Boolean To (0,1)(Boolean=FALSE) -> (0, 1=w792:i16)
                  n704 = Boolean To (0,1)(Boolean=FALSE) -> (0, 1=w790:i16)
                  n705 = Boolean To (0,1)(Boolean=TRUE) -> (0, 1=w791:i16)
                  n706 = Boolean To (0,1)(Boolean=FALSE) -> (0, 1=w789:i16)
                  n707 = Boolean To (0,1)(Boolean=FALSE) -> (0, 1=w788:i16)
                  n708 = local write "Pin2"(w792) -> ()
                  n709 = local write "Pin4"(w790) -> ()
                  n710 = local write "Pin5"(w789) -> ()
                  n711 = local write "Pin3"(w791) -> ()
                  n712 = local write "Pin6"(w788) -> ()
                  n713 = Wait (ms)(milliseconds to wait=u32 3000 ("millisecond timer value")) -> ()  [unwired: 1 out]
                  n714 = local write "Led 1"(FALSE ("Led 1")) -> ()
                  n715 = local write "Led 3"(FALSE ("Led 3")) -> ()
                  n716 = local write "Led 2"(TRUE ("Led 2")) -> ()
                  n717 = local write "Led 4"(FALSE ("Led 4")) -> ()
                  n718 = local write "Led 5"(FALSE ("Led 5")) -> ()
                }
                frame 5 {
                  n719 = Boolean To (0,1)(Boolean=FALSE) -> (0, 1=w808:i16)
                  n720 = Boolean To (0,1)(Boolean=FALSE) -> (0, 1=w806:i16)
                  n721 = Boolean To (0,1)(Boolean=FALSE) -> (0, 1=w807:i16)
                  n722 = Boolean To (0,1)(Boolean=FALSE) -> (0, 1=w805:i16)
                  n723 = Boolean To (0,1)(Boolean=TRUE) -> (0, 1=w804:i16)
                  n724 = local write "Pin2"(w808) -> ()
                  n725 = local write "Pin4"(w806) -> ()
                  n726 = local write "Pin5"(w805) -> ()
                  n727 = local write "Pin3"(w807) -> ()
                  n728 = local write "Pin6"(w804) -> ()
                  n729 = Wait (ms)(milliseconds to wait=u32 3000 ("millisecond timer value")) -> ()  [unwired: 1 out]
                  n730 = local write "Led 1"(FALSE ("Led 1")) -> ()
                  n731 = local write "Led 3"(FALSE ("Led 3")) -> ()
                  n732 = local write "Led 2"(FALSE ("Led 2")) -> ()
                  n733 = local write "Led 4"(FALSE ("Led 4")) -> ()
                  n734 = local write "Led 5"(TRUE ("Led 5")) -> ()
                }
                frame 6 {
                  n735 = Boolean To (0,1)(Boolean=FALSE) -> (0, 1=w824:i16)
                  n736 = Boolean To (0,1)(Boolean=FALSE) -> (0, 1=w822:i16)
                  n737 = Boolean To (0,1)(Boolean=FALSE) -> (0, 1=w823:i16)
                  n738 = Boolean To (0,1)(Boolean=FALSE) -> (0, 1=w821:i16)
                  n739 = Boolean To (0,1)(Boolean=FALSE) -> (0, 1=w820:i16)
                  n740 = local write "Pin2"(w824) -> ()
                  n741 = local write "Pin4"(w822) -> ()
                  n742 = local write "Pin5"(w821) -> ()
                  n743 = local write "Pin3"(w823) -> ()
                  n744 = local write "Pin6"(w820) -> ()
                  n745 = Wait (ms)(milliseconds to wait=u32 3000 ("millisecond timer value")) -> ()  [unwired: 1 out]
                  n746 = local write "Led 1"(FALSE ("Led 1")) -> ()
                  n747 = local write "Led 3"(FALSE ("Led 3")) -> ()
                  n748 = local write "Led 2"(FALSE ("Led 2")) -> ()
                  n749 = local write "Led 4"(FALSE ("Led 4")) -> ()
                  n750 = local write "Led 5"(FALSE ("Led 5")) -> ()
                }
                frame 7 {
                  n751 = Boolean To (0,1)(Boolean=FALSE) -> (0, 1=w840:i16)
                  n752 = Boolean To (0,1)(Boolean=FALSE) -> (0, 1=w838:i16)
                  n753 = Boolean To (0,1)(Boolean=FALSE) -> (0, 1=w839:i16)
                  n754 = Boolean To (0,1)(Boolean=FALSE) -> (0, 1=w837:i16)
                  n755 = Boolean To (0,1)(Boolean=TRUE) -> (0, 1=w836:i16)
                  n756 = local write "Pin2"(w840) -> ()
                  n757 = local write "Pin4"(w838) -> ()
                  n758 = local write "Pin5"(w837) -> ()
                  n759 = local write "Pin3"(w839) -> ()
                  n760 = local write "Pin6"(w836) -> ()
                  n761 = Wait (ms)(milliseconds to wait=u32 3000 ("millisecond timer value")) -> ()  [unwired: 1 out]
                  n762 = local write "Led 1"(FALSE ("Led 1")) -> ()
                  n763 = local write "Led 3"(FALSE ("Led 3")) -> ()
                  n764 = local write "Led 2"(FALSE ("Led 2")) -> ()
                  n765 = local write "Led 4"(FALSE ("Led 4")) -> ()
                  n766 = local write "Led 5"(TRUE ("Led 5")) -> ()
                }
                frame 8 {
                  n767 = Boolean To (0,1)(Boolean=FALSE) -> (0, 1=w856:i16)
                  n768 = Boolean To (0,1)(Boolean=TRUE) -> (0, 1=w854:i16)
                  n769 = Boolean To (0,1)(Boolean=FALSE) -> (0, 1=w855:i16)
                  n770 = Boolean To (0,1)(Boolean=FALSE) -> (0, 1=w853:i16)
                  n771 = Boolean To (0,1)(Boolean=FALSE) -> (0, 1=w852:i16)
                  n772 = local write "Pin2"(w856) -> ()
                  n773 = local write "Pin4"(w854) -> ()
                  n774 = local write "Pin5"(w853) -> ()
                  n775 = local write "Pin3"(w855) -> ()
                  n776 = local write "Pin6"(w852) -> ()
                  n777 = Wait (ms)(milliseconds to wait=u32 3000 ("millisecond timer value")) -> ()  [unwired: 1 out]
                  n778 = local write "Led 1"(FALSE ("Led 1")) -> ()
                  n779 = local write "Led 3"(TRUE ("Led 3")) -> ()
                  n780 = local write "Led 2"(FALSE ("Led 2")) -> ()
                  n781 = local write "Led 4"(FALSE ("Led 4")) -> ()
                  n782 = local write "Led 5"(FALSE ("Led 5")) -> ()
                }
                frame 9 {
                  n783 = Boolean To (0,1)(Boolean=FALSE) -> (0, 1=w872:i16)
                  n784 = Boolean To (0,1)(Boolean=FALSE) -> (0, 1=w870:i16)
                  n785 = Boolean To (0,1)(Boolean=TRUE) -> (0, 1=w871:i16)
                  n786 = Boolean To (0,1)(Boolean=FALSE) -> (0, 1=w869:i16)
                  n787 = Boolean To (0,1)(Boolean=FALSE) -> (0, 1=w868:i16)
                  n788 = local write "Pin2"(w872) -> ()
                  n789 = local write "Pin4"(w870) -> ()
                  n790 = local write "Pin5"(w869) -> ()
                  n791 = local write "Pin3"(w871) -> ()
                  n792 = local write "Pin6"(w868) -> ()
                  n793 = Wait (ms)(milliseconds to wait=u32 3000 ("millisecond timer value")) -> ()  [unwired: 1 out]
                  n794 = local write "Led 1"(FALSE ("Led 1")) -> ()
                  n795 = local write "Led 3"(FALSE ("Led 3")) -> ()
                  n796 = local write "Led 2"(TRUE ("Led 2")) -> ()
                  n797 = local write "Led 4"(FALSE ("Led 4")) -> ()
                  n798 = local write "Led 5"(FALSE ("Led 5")) -> ()
                }
                frame 10 {
                  n799 = Boolean To (0,1)(Boolean=FALSE) -> (0, 1=w888:i16)
                  n800 = Boolean To (0,1)(Boolean=FALSE) -> (0, 1=w886:i16)
                  n801 = Boolean To (0,1)(Boolean=FALSE) -> (0, 1=w887:i16)
                  n802 = Boolean To (0,1)(Boolean=TRUE) -> (0, 1=w885:i16)
                  n803 = Boolean To (0,1)(Boolean=FALSE) -> (0, 1=w884:i16)
                  n804 = local write "Pin2"(w888) -> ()
                  n805 = local write "Pin4"(w886) -> ()
                  n806 = local write "Pin5"(w885) -> ()
                  n807 = local write "Pin3"(w887) -> ()
                  n808 = local write "Pin6"(w884) -> ()
                  n809 = Wait (ms)(milliseconds to wait=u32 3000 ("millisecond timer value")) -> ()  [unwired: 1 out]
                  n810 = local write "Led 1"(FALSE ("Led 1")) -> ()
                  n811 = local write "Led 3"(FALSE ("Led 3")) -> ()
                  n812 = local write "Led 2"(FALSE ("Led 2")) -> ()
                  n813 = local write "Led 4"(TRUE ("Led 4")) -> ()
                  n814 = local write "Led 5"(FALSE ("Led 5")) -> ()
                }
                frame 11 {
                  n815 = Boolean To (0,1)(Boolean=TRUE) -> (0, 1=w904:i16)
                  n816 = Boolean To (0,1)(Boolean=FALSE) -> (0, 1=w902:i16)
                  n817 = Boolean To (0,1)(Boolean=FALSE) -> (0, 1=w903:i16)
                  n818 = Boolean To (0,1)(Boolean=FALSE) -> (0, 1=w901:i16)
                  n819 = Boolean To (0,1)(Boolean=FALSE) -> (0, 1=w900:i16)
                  n820 = local write "Pin2"(w904) -> ()
                  n821 = local write "Pin4"(w902) -> ()
                  n822 = local write "Pin5"(w901) -> ()
                  n823 = local write "Pin3"(w903) -> ()
                  n824 = local write "Pin6"(w900) -> ()
                  n825 = Wait (ms)(milliseconds to wait=u32 3000 ("millisecond timer value")) -> ()  [unwired: 1 out]
                  n826 = local write "Led 1"(TRUE ("Led 1")) -> ()
                  n827 = local write "Led 3"(FALSE ("Led 3")) -> ()
                  n828 = local write "Led 2"(FALSE ("Led 2")) -> ()
                  n829 = local write "Led 4"(FALSE ("Led 4")) -> ()
                  n830 = local write "Led 5"(FALSE ("Led 5")) -> ()
                }
                frame 12 {
                  n831 = Boolean To (0,1)(Boolean=FALSE) -> (0, 1=w921:i16)
                  n832 = Boolean To (0,1)(Boolean=FALSE) -> (0, 1=w919:i16)
                  n833 = Boolean To (0,1)(Boolean=FALSE) -> (0, 1=w920:i16)
                  n834 = Boolean To (0,1)(Boolean=FALSE) -> (0, 1=w918:i16)
                  n835 = Boolean To (0,1)(Boolean=FALSE) -> (0, 1=w917:i16)
                  n836 = Wait (ms)(milliseconds to wait=u32 3000 ("millisecond timer value")) -> ()  [unwired: 1 out]
                  n837 = local write "Pin2"(w921) -> ()
                  n838 = local write "Pin4"(w919) -> ()
                  n839 = local write "Pin5"(w918) -> ()
                  n840 = local write "Pin3"(w920) -> ()
                  n841 = local write "Pin6"(w917) -> ()
                  n842 = local write "Contenido"(-1.0 ("Contenido")) -> ()
                  n843 = local write "Led 1"(FALSE ("Led 1")) -> ()
                  n844 = local write "Led 3"(FALSE ("Led 3")) -> ()
                  n845 = local write "Led 2"(FALSE ("Led 2")) -> ()
                  n846 = local write "Led 4"(FALSE ("Led 4")) -> ()
                  n847 = local write "Led 5"(FALSE ("Led 5")) -> ()
                }
              }
            }
          }
          n848 = call-poly <vilib>:"Digital Read.vi"("Error In"=w88, "DI Channel"=u8 3, "LINX Resource"=w97) -> ("Error Out"=w87:errorcluster, "LINX Resource"=w96:T2)  [unwired: 6 in, 1 out]
          n849 = local read "Led 2"() -> (w77:bool)
          n850 = local write "Pin3"(w80) -> ()
          n851 = call-poly <vilib>:"Digital Write.vi"("Error In"=w87, "Output Value"=w77, "DO Channel"=w80, "LINX Resource"=w96) -> ("Error Out"=w86:errorcluster, "LINX Resource"=w95:T2)  [unwired: 6 in]
          n852 = call-poly <vilib>:"Digital Read.vi"("Error In"=w86, "DI Channel"=u8 4, "LINX Resource"=w95) -> ("Error Out"=w85:errorcluster, "LINX Resource"=w94:T2)  [unwired: 6 in, 1 out]
          n853 = local read "Led 3"() -> (w76:bool)
          n854 = local write "Pin4"(w75) -> ()
          n855 = call-poly <vilib>:"Digital Write.vi"("Error In"=w85, "Output Value"=w76, "DO Channel"=w75, "LINX Resource"=w94) -> ("Error Out"=w84:errorcluster, "LINX Resource"=w93:T2)  [unwired: 6 in]
          n856 = call-poly <vilib>:"Digital Read.vi"("Error In"=w84, "DI Channel"=u8 5, "LINX Resource"=w93) -> ("Error Out"=w83:errorcluster, "LINX Resource"=w92:T2)  [unwired: 6 in, 1 out]
          n857 = local write "Pin5"(w74) -> ()
          n858 = local read "Led 4"() -> (w73:bool)
          n859 = call-poly <vilib>:"Digital Write.vi"("Error In"=w83, "Output Value"=w73, "DO Channel"=w74, "LINX Resource"=w92) -> ("Error Out"=w82:errorcluster, "LINX Resource"=w91:T2)  [unwired: 6 in]
          n860 = call-poly <vilib>:"Digital Read.vi"("Error In"=w82, "DI Channel"=u8 6, "LINX Resource"=w91) -> ("Error Out"=w81:errorcluster, "LINX Resource"=w90:T2)  [unwired: 6 in, 1 out]
          n861 = local write "Pin6"(w71) -> ()
          n862 = local read "Led 5"() -> (w72:bool)
          n863 = call-poly <vilib>:"Digital Write.vi"("Error In"=w81, "Output Value"=w72, "DO Channel"=w71, "LINX Resource"=w90) -> ("Error Out"=w69:errorcluster, "LINX Resource"=w70:T2)  [unwired: 6 in]
        }
        n864 = local write "Tab Control"(enum32{"Inicio", "Sistema"}."Sistema" ("Tab Control")) -> ()
        n865 = call <vilib>:"Close.vi"("Error In"=w47, "LINX Resource"=w48) -> ("Error Out"=w55:errorcluster)  [unwired: 9 in]
        n866 = call <vilib>:"Simple Error Handler.vi"("error in (no error)"=w55) -> ()  [unwired: 4 in, 5 out]
        "Contenido" <- 0.0 ("Contenido")
        "Pin2" <- 0.0 ("Pin2")
        "Pin3" <- 0.0 ("Pin3")
        "Pin4" <- 0.0 ("Pin4")
        "Pin5" <- 0.0 ("Pin5")
        "Pin6" <- 0.0 ("Pin6")
      }
      frame #2 {
        n867 = local write "Tab Control"(enum32{"Inicio", "Sistema"}."Inicio" ("Tab Control")) -> ()
      }
    }
  }
  n868 = local write "Usuario"("" ("Usuario")) -> ()
  n869 = local write "Contraseña"("" ("Contraseña")) -> ()
